vi "FTW-CodeGen-UpdateStateWithRef.vi"(0 "Old State":variant, 5 "XRef":refnum<vi>, 7 "Version":T1) -> (4 "State Out":T2, 6 "Reply":string[](array[string]), 8 "Is Good?":bool)   [LabVIEW 2015, in "FTW-SQLite-Fetch.xnode"]
uses:
  FTW-SQLite-Fetch.xnode
  FTW-CodeGen-State.ctl
panel:
  # "Inputs"
  # "Outputs"
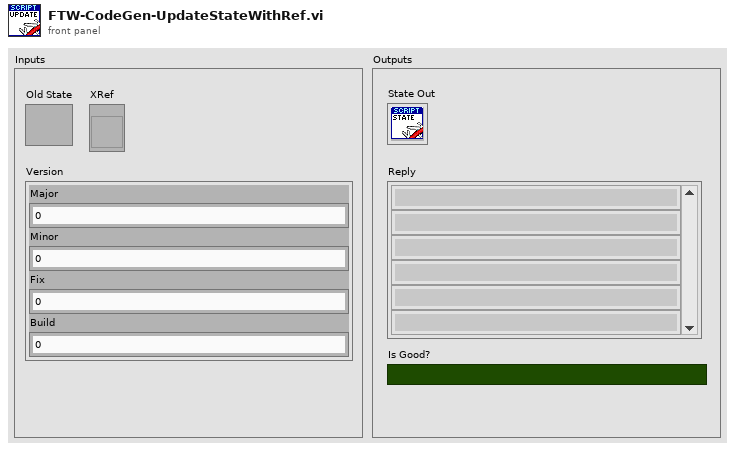
[diagram p1: front panel]
types:
  T1 = cluster{"Major":u16, "Minor":u16, "Fix":u16, "Build":u16}
  T2 = typedef "FTW-SQLite-Fetch.xnode/FTW-CodeGen-State.ctl" = cluster{"Dummy":i32}
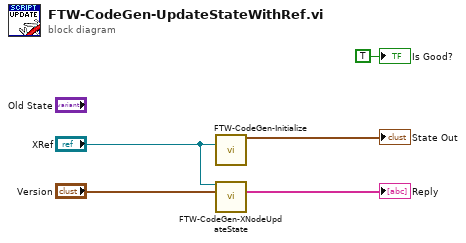
[diagram p0: block diagram]
diagram:
  n1 = call "FTW-CodeGen-Initialize.vi"("XRef"="XRef") -> ("State Out"=→"State Out":T2)  [unwired: 14 in]
  n2 = call "FTW-CodeGen-XNodeUpdateState.vi"("XRef"="XRef", "Version"="Version") -> ("Reply"=→"Reply":string[])  [unwired: 13 in]
  "Is Good?" <- TRUE ("Is Good?")
